vi "Periodic Tasks.vi"(8 "error in":errorcluster) -> ()   [LabVIEW 2013]
doc: "This VI runs in parallel to other tasks. It can contain as many user-defined periodic loops as you need. These can carry out PID or other sorts of timed response."
uses:
  <vilib>/Rock Robotics/SystemInterfaces/Utilities/FPGA_UtilitiesLED Source.ctl
  <vilib>/Rock Robotics/SystemInterfaces/Utilities/FPGA_UtilitiesLED State.ctl
  PressureSensorAction.ctl
  PassType.ctl
  PassState.ctl
  <vilib>/Rock Robotics/WPI/Compressor/WPI_CompressorGetSetRefNum.vi
  Robot Global Data.vi
panel:
  out "Drive Loop Iterations":i32
  out "Main Loop Interations":i32
  out "Pressure Sensor Iterations":i32
  out "Pressure Sensor Loop Time":u32
  out "Handler Iterations":i32
  in  "HalfDriveScalar":dbl=0.6
  out "Handler Skipped Data?":bool
  out "Main Loop Time":u32
  out "Handler Loop Time":u32
  out "Drive Loop Time":u32
  out "HandleInputElements":i32
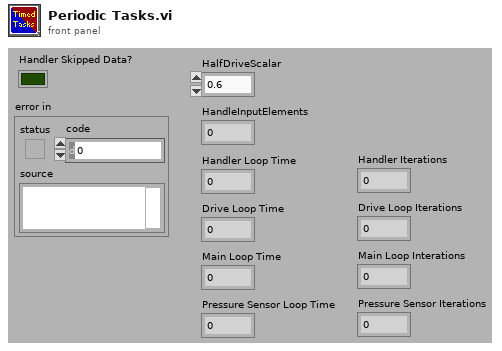
[diagram p1: front panel]
types:
  T1 = typedef "TeleopInstruction.ctl" = cluster{"cDriveLeft":dbl, "cDriveRight":dbl, "cAutoDistance":bool, "cHalfDrive":bool, "cStraightDrive":bool, "cReverseDrive":bool, "cSonicShifter":bool, "cRoller":dbl, "cCollector":dbl, "cServo":dbl, "cPass":bool, "cCatch":bool, "cCollectorWrap":bool, "cShooter":bool, "cClapperIn":bool, "cClapperOut":bool, "cFiringPneumatic":bool, "cKickerPneumatic":bool, "cRollerPneumatic":bool, "TeleopID":i32}
  T2 = typedef "DriveInstruction.ctl" = cluster{"DriveData":T3, "Subsystem":T4, "Action":T5}
  T3 = typedef "DriveData.ctl" = cluster{"cDriveLeft":dbl, "cDriveRight":dbl, "cHalfDrive":bool, "cStraightDrive":bool, "cReverseDrive":bool}
  T4 = typedef "QueueSubsystem.ctl" = enum16{"Drive", "SonicShifter", "Kicker", "FiringPneumatic", "RollerPneumatic", "Clapper", "RollerMotor", "CollectorMotor", "Servo", "ShooterWrapper", "CollectorWrapper", "CatcherWrapper", "AutoDistance", "PassWrapper"}
  T5 = typedef "TankDriveAction.ctl" = enum16{"Init", "LinearDrive", "SetValue", "Disable"}
  T6 = typedef "FPGA_UtilitiesLED State.ctl" = enum16{"Off", "On", "Toggle"}
  T7 = typedef "FPGA_UtilitiesLED Source.ctl" = enum16{"User LED", "FPGA LED"}
  T8 = typedef "PassType.ctl" = enum16{"Ground", "Elevated"}
  T9 = typedef "PassState.ctl" = enum16{"Pass", "Stop"}
  T10 = typedef "QueueInstruction.ctl" = cluster{"Data":variant, "Subsystem":T4, "Action":T11}
  T11 = typedef "QueueAction.ctl" = enum16{"Init", "SetValue", "Disable"}
  T12 = typedef "DoubleSolenoidAction.ctl" = enum16{"Init", "Middle", "In", "Out"}
  T13 = typedef "RollerAction.ctl" = enum16{"Init", "Off", "Forward", "Reverse"}
  T14 = typedef "CollectorWrapAction.ctl" = enum16{"PreCollect", "Collect", "Stop"}
  T15 = typedef "ServoAction.ctl" = enum16{"Init", "SetAngle", "GetAngle", "Lower", "Raise", "Disable"}
  T16 = typedef "ShooterWrapperAction.ctl" = enum16{"Init", "CollectorDown", "CollectorUp"}
  T17 = typedef "CatchAction.ctl" = enum16{"PreCatch", "Catch", "Stop"}
  T18 = typedef "PressureSensorAction.ctl" = enum16{"Init", "ReadValue", "Disable"}
  T19 = typedef "WPI_CompressorDevRef.ctl" = cluster{"DevStatus":errorcluster, "DigitalInputDevRef":T20, "RelayDevRef":T23}
  T20 = typedef "WPI_DigitalInputDevRef.ctl" = cluster{"DevStatus":errorcluster, "DIO Channel":T21, "Digital Module":T22}
  T21 = typedef "FPGA_DIOChannel.ctl" = enum8{"DIO 1", "DIO 2", "DIO 3", "DIO 4", "DIO 5", "DIO 6", "DIO 7", "DIO 8", "DIO 9", "DIO 10", "DIO 11", "DIO 12", "DIO 13", "DIO 14", "Invalid"}
  T22 = typedef "FPGA_TypedefDigitalModule.ctl" = enum16{"Digital Module 1", "Digital Module 2"}
  T23 = typedef "WPI_RelayDevRef.ctl" = cluster{"DevStatus":errorcluster, "Relay Channel":T24, "Digital Module":T22, "Relay Direction":T25}
  T24 = typedef "FPGA_DIORelayChannel.ctl" = enum8{"Relay 1", "Relay 2", "Relay 3", "Relay 4", "Relay 5", "Relay 6", "Relay 7", "Relay 8", "Invalid"}
  T25 = typedef "WPI_RelayDirection.ctl" = enum16{"Both directions", "Forward only", "Reverse only"}
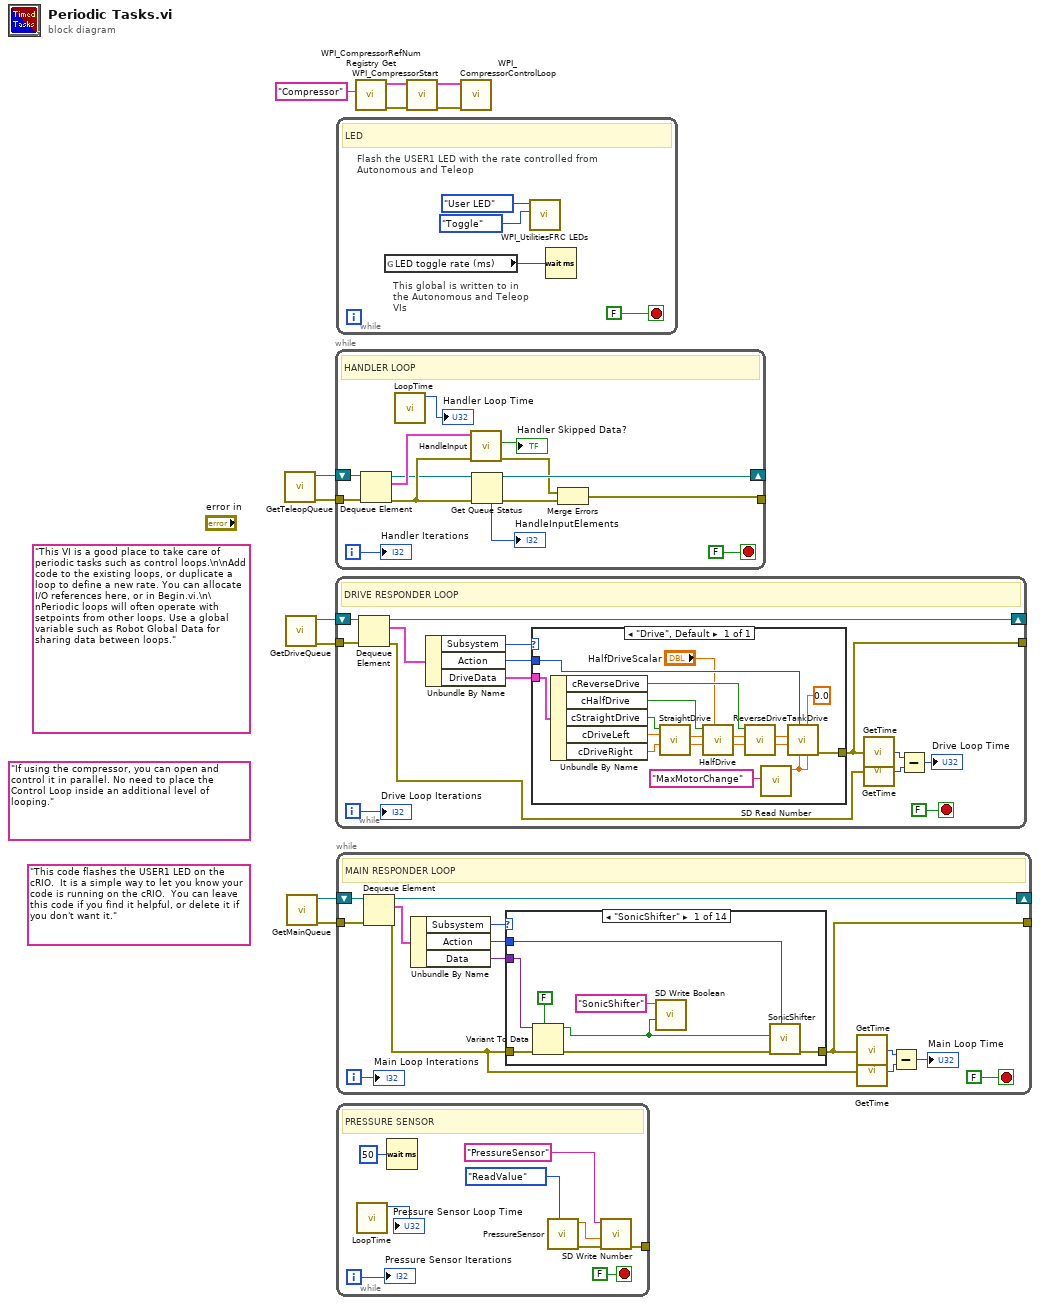
[diagram p0: block diagram]
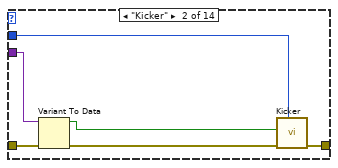
[diagram p2: hidden frame]
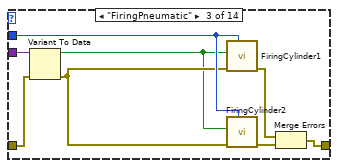
[diagram p3: hidden frame]
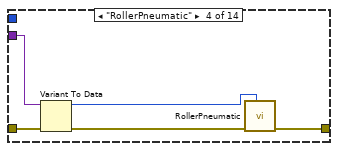
[diagram p4: hidden frame]
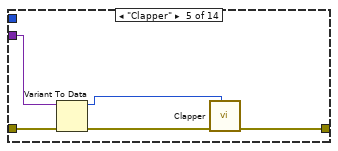
[diagram p5: hidden frame]
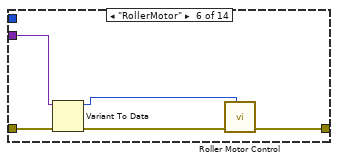
[diagram p6: hidden frame]
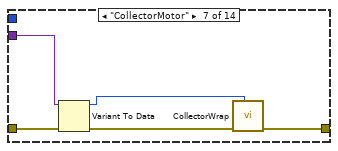
[diagram p7: hidden frame]
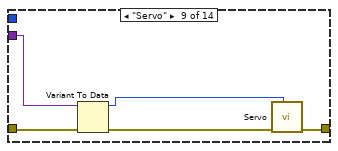
[diagram p9: hidden frame]
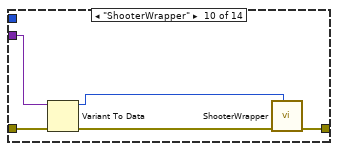
[diagram p10: hidden frame]
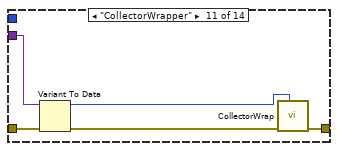
[diagram p11: hidden frame]
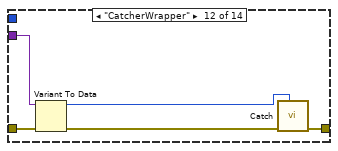
[diagram p12: hidden frame]
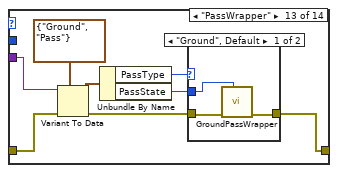
[diagram p13: hidden frame]
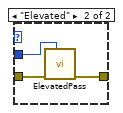
[diagram p14: hidden frame]
diagram:
  (unwired) "If using the compressor, you can open and control it in parallel. No need to place the Control Loop inside an additional level of looping."
  (unwired) "This code flashes the USER1 LED on the cRIO.  It is a simple way to let you know your code is running on the cRIO.  You can leave this code if you find it helpful, or delete it if you don't want it."
  (unwired) "This VI is a good place to take care of periodic tasks such as control loops.\n\nAdd code to the existing loops, or duplicate a loop to define a new rate. You can allocate I/O references here, or in Begin.vi.\n\nPeriodic loops will often operate with setpoints from other loops. Use a global variable such as Robot Global Data for sharing data between loops."
  n1 = call "GetTeleopQueue.vi"() -> ("error out"=w5:errorcluster, "queue out"=w6:refnum<queue>)  [unwired: 10 in]
  n2 = call "GetDriveQueue.vi"() -> ("error out"=w4:errorcluster, "queue out"=w3:refnum<queue>)  [unwired: 10 in]
  n3 = call "GetMainQueue.vi"() -> ("error out"=w1:errorcluster, "queue out"=w2:refnum<queue>)  [unwired: 10 in]
  n4 = while {
    shift-right: [w23] -> _
    shift-left: w6 -> [w24]
    tunnel: w5 -> [w25]
    tunnel: [w16] -> _
    i -> [w12]
    stop <- FALSE stop-if-true
    # "HANDLER LOOP"
    n5 = Dequeue Element(queue=w24, error in (no error)=w25) -> (queue out=w19:refnum<queue>, element=w21:T1, error out=w20:errorcluster)  [unwired: 1 in, 1 out]
    n6 = call "LoopTime.vi"() -> ("LoopTime"=→"Handler Loop Time":u32)  [unwired: 11 in]
    n7 = call "HandleInput.vi"("error in (no error)"=w20, "TeleopInstruction"=w21) -> ("error out"=w17:errorcluster, "SkippedData?"=→"Handler Skipped Data?":bool)  [unwired: 7 in, 1 out]
    n8 = Get Queue Status(queue=w19, error in (no error)=w20) -> (queue out=w23:refnum<queue>, error out=w18:errorcluster, # elements in queue=→"HandleInputElements":i32)  [unwired: 1 in, 5 out]
    n9 = Merge Errors(w17, w18) -> (w16:errorcluster)
    "Handler Iterations" <- w12
  }
  n10 = while {
    shift-right: [w38] -> _
    shift-left: w3 -> [w39]
    tunnel: w4 -> [w37]
    tunnel: [w30] -> _
    i -> [w26]
    stop <- FALSE stop-if-true
    # "DRIVE RESPONDER LOOP"
    n11 = Dequeue Element(queue=w39, error in (no error)=w37) -> (queue out=w38:refnum<queue>, element=w36:T2, error out=w31:errorcluster)  [unwired: 1 in, 1 out]
    n12 = Unbundle By Name(w36) -> ("Subsystem"=w35:T4, "Action"=w34:T5, "DriveData"=w33:T3)
    n13 = case shown="\"Drive\", Default" w35 {
      tunnel: w34 -> [w57]
      tunnel: w33 -> [w55]
      tunnel: [w43] -> w30
      frame "Drive", Default {
        n14 = Unbundle By Name(w55) -> ("cReverseDrive"=w46:bool, "cHalfDrive"=w45:bool, "cStraightDrive"=w44:bool, "cDriveLeft"=w54:dbl, "cDriveRight"=w53:dbl)
        n15 = call "StraightDrive.vi"("RightDrive in"=w53, "LeftDrive in"=w54, "StraightDrive"=w44) -> ("RightDrive out"=w51:dbl, "LeftDrive out"=w52:dbl)  [unwired: 7 in]
        n16 = call "HalfDrive.vi"("Scaler"="HalfDriveScalar", "RightDrive in"=w51, "LeftDrive in"=w52, "HalfDrive"=w45) -> ("RightDrive out"=w49:dbl, "LeftDrive out"=w50:dbl)  [unwired: 6 in]
        n17 = call "ReverseDrive.vi"("Right"=w49, "Left"=w50, "cReverseDrive"=w46) -> ("Right"=w47:dbl, "Left"=w48:dbl)  [unwired: 7 in]
        n18 = call <vilib>:"SD Read Number.vi"("Name"="MaxMotorChange") -> ("Numeric"=w40:dbl)  [unwired: 8 in, 2 out]
        n19 = call "TankDrive.vi"("MaxMotorChangeForward"=w40, "Cutoff"=0.0, "MaxMotorChangeBackward"=w40, "DriveAction"=w57, "RightDesired"=w47, "LeftDesired"=w48) -> ("error out"=w43:errorcluster)  [unwired: 4 in, 1 out]
      }
    }
    n20 = call "GetTime.vi"("error in"=w30) -> ("Time"=w28:u32)
    n21 = call "GetTime.vi"("error in"=w31) -> ("Time"=w29:u32)
    n22 = Subtract(x=w28, y=w29) -> (x-y=→"Drive Loop Time":u32)
    "Drive Loop Iterations" <- w26
  }
  n23 = while {
    stop <- FALSE stop-if-true
    # "This global is written to in the Autonomous and Teleop VIs"
    # "Flash the USER1 LED with the rate controlled from Autonomous and Teleop"
    # "LED"
    n24 = global read "Robot Global Data.vi" "LED toggle rate (ms)"() -> (w58:u32)
    n25 = call <vilib>:"WPI_UtilitiesFRC LEDs.vi"("State"=FPGA_UtilitiesLED_State."Toggle", "LED Type"=FPGA_UtilitiesLED_Source."User LED") -> ()  [unwired: 1 in, 9 out]
    n26 = Wait (ms)(milliseconds to wait=w58) -> ()  [unwired: 1 out]
  }
  n27 = while {
    shift-right: [w73] -> _
    shift-left: w2 -> [w74]
    tunnel: w1 -> [w75]
    tunnel: [w67] -> _
    i -> [w62]
    stop <- FALSE stop-if-true
    # "MAIN RESPONDER LOOP"
    n28 = Dequeue Element(queue=w74, error in (no error)=w75) -> (queue out=w73:refnum<queue>, element=w72:T10, error out=w63:errorcluster)  [unwired: 1 in, 1 out]
    n29 = Unbundle By Name(w72) -> ("Subsystem"=w71:T4, "Action"=w70:T11, "Data"=w69:variant)
    n30 = case shown="\"SonicShifter\"" w71 {
      tunnel: [w79 w89 w94 w102 w107 w112 w114 w118 w123 w128 w133 w138 w146 _] -> w67
      tunnel: w63 -> [w81 w88 w92 w99 w106 w110 w117 w118 w121 w127 w132 w137 w143 _]
      tunnel: w70 -> [w83 w84 w96 _ _ _ _ _ _ _ _ _ _ _]
      tunnel: w69 -> [w82 w86 w97 w101 w104 w111 w116 _ w120 w125 w129 w134 w145 _]
      frame "SonicShifter" {
        n31 = Variant To Data(error in=w81, type=FALSE, Variant=w82) -> (data=w76:bool, error out=w80:errorcluster)
        n32 = call <vilib>:"SD Write Boolean.vi"("Boolean"=w76, "Name"="SonicShifter") -> ()  [unwired: 8 in, 2 out]
        n33 = call "SonicShifter.vi"("Action"=w83, "error in (no error)"=w80, "Actuate?"=w76) -> ("error out"=w79:errorcluster)  [unwired: 8 in]
      }
      frame "Kicker" {
        n34 = Variant To Data(error in=w88, Variant=w86) -> (data=w85:bool, error out=w87:errorcluster)  [unwired: 1 in]
        n35 = call "Kicker.vi"("Action"=w84, "error in (no error)"=w87, "Actuate?"=w85) -> ("error out"=w89:errorcluster)  [unwired: 8 in]
      }
      frame "FiringPneumatic" {
        n36 = Variant To Data(error in=w92, Variant=w97) -> (data=w90:bool, error out=w91:errorcluster)  [unwired: 1 in]
        n37 = call "FiringCylinder1.vi"("Action"=w96, "error in (no error)"=w91, "Actuate?"=w90) -> ("error out"=w93:errorcluster)  [unwired: 8 in]
        n38 = call "FiringCylinder2.vi"("Action"=w96, "error in (no error)"=w91, "Actuate?"=w90) -> ("error out"=w95:errorcluster)  [unwired: 8 in]
        n39 = Merge Errors(w93, w95) -> (w94:errorcluster)
      }
      frame "RollerPneumatic" {
        n40 = Variant To Data(error in=w99, Variant=w101) -> (data=w100:T12, error out=w98:errorcluster)  [unwired: 1 in]
        n41 = call "RollerPneumatic.vi"("State"=w100, "Error in"=w98) -> ("Error out"=w102:errorcluster)  [unwired: 9 in]
      }
      frame "Clapper" {
        n42 = Variant To Data(error in=w106, Variant=w104) -> (data=w103:T12, error out=w105:errorcluster)  [unwired: 1 in]
        n43 = call "Clapper.vi"("State"=w103, "Error in"=w105) -> ("Error out"=w107:errorcluster)  [unwired: 9 in]
      }
      frame "RollerMotor" {
        n44 = Variant To Data(error in=w110, Variant=w111) -> (data=w108:T13, error out=w109:errorcluster)  [unwired: 1 in]
        n45 = call "Roller Motor Control.vi"("Action"=w108, "Error in"=w109) -> ("Error out"=w112:errorcluster)  [unwired: 9 in]
      }
      frame "CollectorMotor" {
        n46 = Variant To Data(error in=w117, Variant=w116) -> (data=w113:T14, error out=w115:errorcluster)  [unwired: 1 in]
        n47 = call "CollectorWrap.vi"("Action"=w113, "error in"=w115) -> ("error out"=w114:errorcluster)  [unwired: 8 in, 1 out]
      }
      frame "Drive" {
        # "\"Should\" be handled in drive loop"
      }
      frame "Servo" {
        n48 = Variant To Data(error in=w121, Variant=w120) -> (data=w119:T15, error out=w122:errorcluster)  [unwired: 1 in]
        n49 = call "Servo.vi"("Action"=w119, "error in (no error)"=w122) -> ("error out"=w123:errorcluster)  [unwired: 8 in, 1 out]
      }
      frame "ShooterWrapper" {
        n50 = Variant To Data(error in=w127, Variant=w125) -> (data=w124:T16, error out=w126:errorcluster)  [unwired: 1 in]
        n51 = call "ShooterWrapper.vi"("Action"=w124, "error in"=w126) -> ("error out"=w128:errorcluster)  [unwired: 8 in]
      }
      frame "CollectorWrapper" {
        n52 = Variant To Data(error in=w132, Variant=w129) -> (data=w130:T14, error out=w131:errorcluster)  [unwired: 1 in]
        n53 = call "CollectorWrap.vi"("Action"=w130, "error in"=w131) -> ("error out"=w133:errorcluster)  [unwired: 8 in, 1 out]
      }
      frame "CatcherWrapper" {
        n54 = Variant To Data(error in=w137, Variant=w134) -> (data=w135:T17, error out=w136:errorcluster)  [unwired: 1 in]
        n55 = call "Catch.vi"("Action"=w135, "error in (no error)"=w136) -> ("error out"=w138:errorcluster)  [unwired: 9 in]
      }
      frame "PassWrapper" {
        n56 = Variant To Data(error in=w143, type=cluster{"PassType":T8, "PassState":T9} {"PassType"=enum."Ground", "PassState"=enum."Pass"}, Variant=w145) -> (data=w141:cluster{"PassType":T8, "PassState":T9}, error out=w142:errorcluster)
        n57 = Unbundle By Name(w141) -> ("PassType"=w140:T8, "PassState"=w139:T9)
        n58 = case shown="\"Ground\", Default" w140 {
          tunnel: [w149 w151] -> w146
          tunnel: w142 -> [w148 w152]
          tunnel: w139 -> [w147 w150]
          frame "Ground", Default {
            n59 = call "GroundPassWrapper.vi"("State"=w147, "error in"=w148) -> ("error out"=w149:errorcluster)  [unwired: 9 in]
          }
          frame "Elevated" {
            n60 = call "ElevatedPass.vi"("PassState"=w150, "error in (no error)"=w152) -> ("error out"=w151:errorcluster)  [unwired: 9 in]
          }
        }
      }
      frame "AutoDistance" {
      }
    }
    n61 = call "GetTime.vi"("error in"=w67) -> ("Time"=w66:u32)
    n62 = call "GetTime.vi"("error in"=w63) -> ("Time"=w65:u32)
    n63 = Subtract(x=w66, y=w65) -> (x-y=→"Main Loop Time":u32)
    "Main Loop Interations" <- w62
  }
  n64 = while {
    tunnel: [w158] -> _
    i -> [w154]
    stop <- FALSE stop-if-true
    # "PRESSURE SENSOR"
    n65 = call "LoopTime.vi"() -> ("LoopTime"=→"Pressure Sensor Loop Time":u32)  [unwired: 11 in]
    n66 = Wait (ms)(milliseconds to wait=u32 50) -> ()  [unwired: 1 out]
    n67 = call "PressureSensor.vi"("Action"=PressureSensorAction."ReadValue") -> ("error out"=w159:errorcluster, "Pressure"=w157:dbl)  [unwired: 9 in]
    n68 = call <vilib>:"SD Write Number.vi"("error in"=w159, "Numeric"=w157, "Name"="PressureSensor") -> ("error out"=w158:errorcluster)  [unwired: 7 in, 1 out]
    "Pressure Sensor Iterations" <- w154
  }
  n69 = call <vilib>:"WPI_CompressorRefNum Registry Get.vi"("refnum name"="Compressor") -> ("error out"=w10:errorcluster, "CompressorDevRef"=w9:T19)  [unwired: 9 in]
  n70 = call <vilib>:"WPI_CompressorStart.vi"("error in (no error)"=w10, "CompressorDevRef"=w9) -> ("error out"=w8:errorcluster, "CompressorDevRef"=w7:T19)  [unwired: 8 in]
  n71 = call <vilib>:"WPI_CompressorControlLoop.vi"("error in (no error)"=w8, "CompressorDevRef"=w7) -> ()  [unwired: 10 in]
